vi "RT Accquistion.vi"(7 "Queue ref":T2, 8 "error in":errorcluster, 10 "UI Data":refnum<notifier>, 11 "Task":T3) -> (0 "error out":errorcluster[](array[cluster]))   [LabVIEW 2022 SP3]
uses:
  <vilib>/DAQmx/read.llb/DAQmx Read (Analog 1D Wfm NChan NSamp).vi
  <vilib>/DAQmx/write.llb/DAQmx Write (Analog 1D DBL NChan 1Samp).vi
  <vilib>/DAQmx/write.llb/DAQmx Write (Digital 1D Bool NChan 1Samp 1Line).vi
  <vilib>/DAQmx/read.llb/DAQmx Read (Digital 1D Wfm NChan NSamp).vi
  Source code/Controls/All Loop Status.ctl
  Source code/Controls/All Queue.ctl
  Source code/Controls/UI Data.ctl
panel:
  in  "notification":T1
  out "TC":waveform(dbl)[](array[waveform])
  out "DI":digitalwaveform[](array[waveform])
  out "AI":waveform(dbl)[](array[waveform])
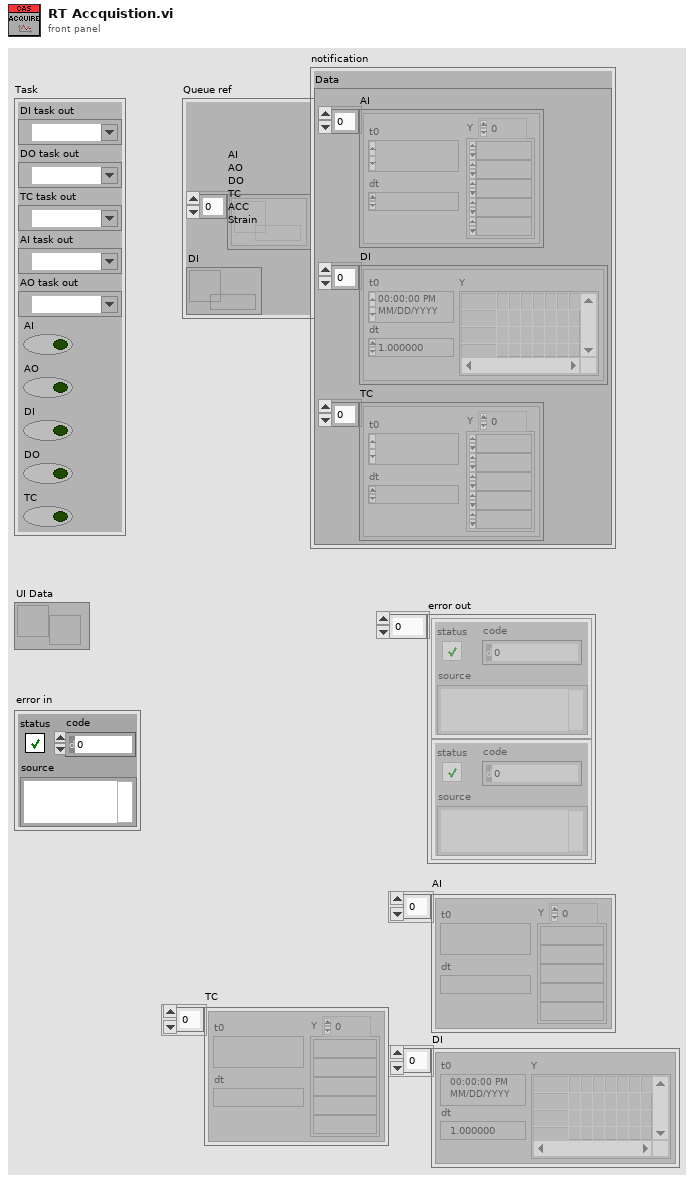
[diagram p1: front panel]
types:
  T1 = typedef "UI Data.ctl" = cluster{"Data":cluster{"AI":waveform(dbl)[], "DI":digitalwaveform[], "TC":waveform(dbl)[]}}
  T2 = typedef "All Queue.ctl" = cluster{"AI\nAO\nDO\nTC\nACC\nStrain":refnum<queue>[], "DI":refnum<queue>}
  T3 = cluster{"DI task out":refnum<k21>, "DO task out":refnum<k21>, "TC task out":refnum<k21>, "AI task out":refnum<k21>, "AO task out":refnum<k21>, "AI":bool, "AO":bool, "DI":bool, "DO":bool, "TC":bool}
  T4 = enum16{"Init", "Read 'All'", "Read 'n'", "Read '1'", "Write '1'", "Write 'n'", "Write 'All'"}
  T5 = typedef "All Loop Status.ctl" = enum16{"AI", "AO", "DI", "DO", "TC", "Strain", "ACC", "RT", "Log"}
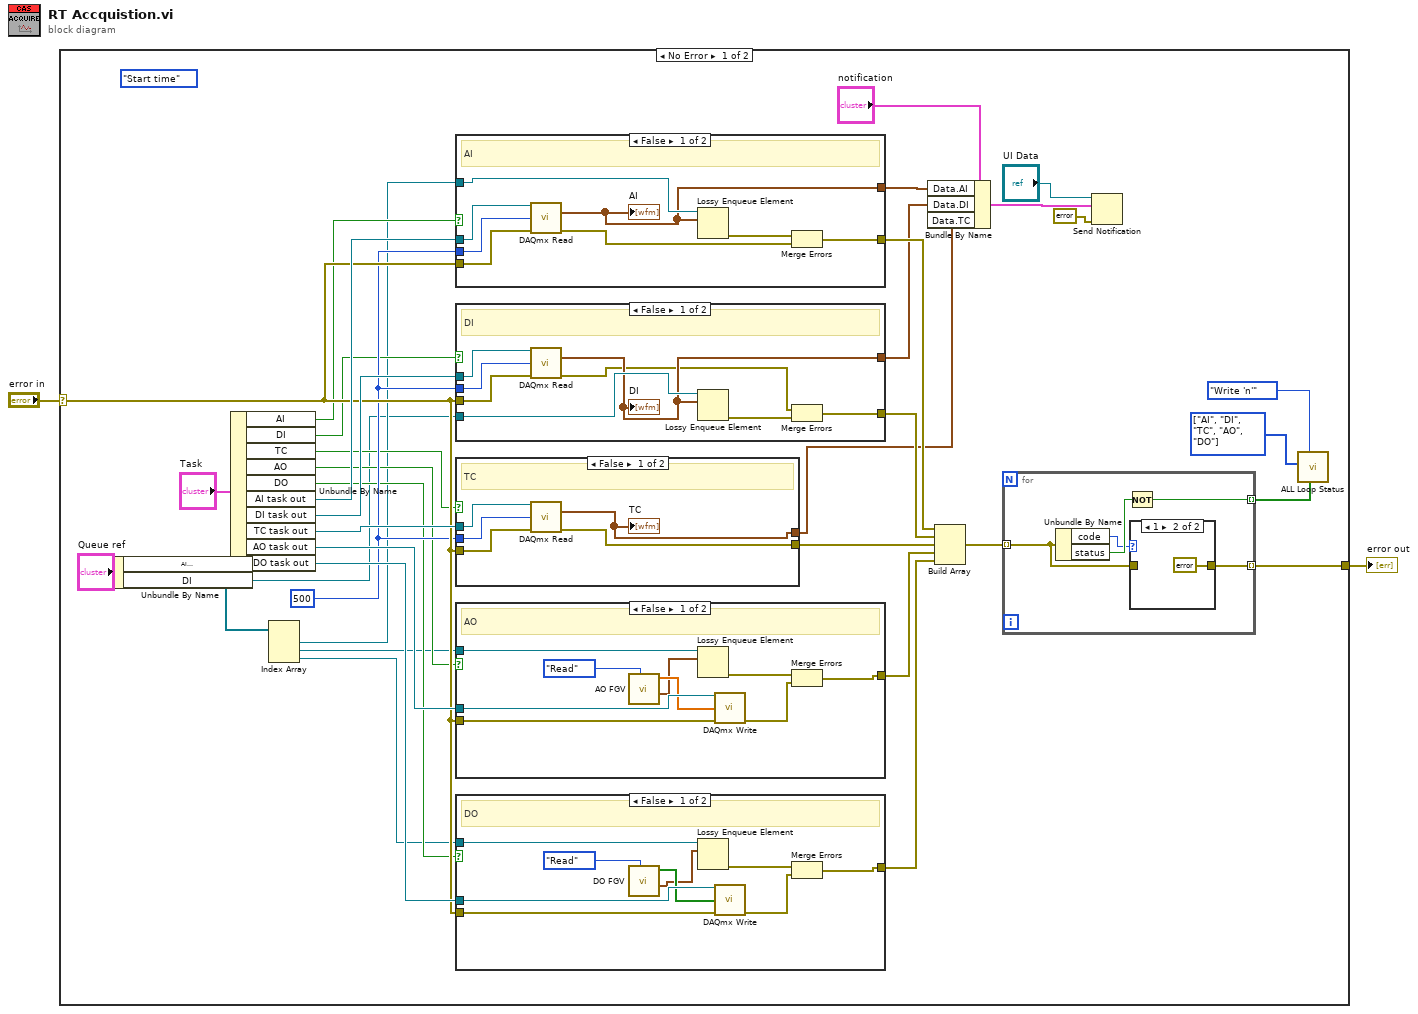
[diagram p0: block diagram]
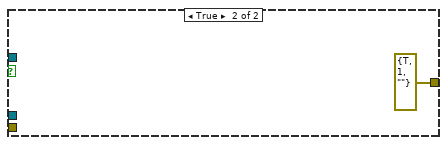
[diagram p3: hidden frame]
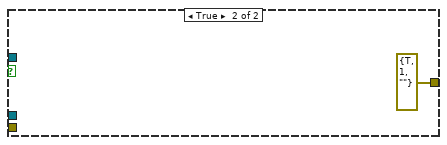
[diagram p4: hidden frame]
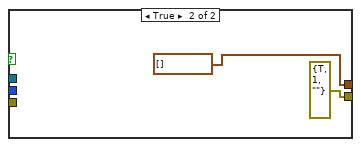
[diagram p5: hidden frame]
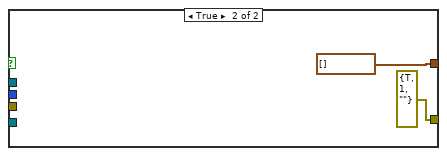
[diagram p6: hidden frame]
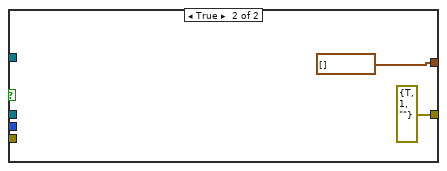
[diagram p7: hidden frame]
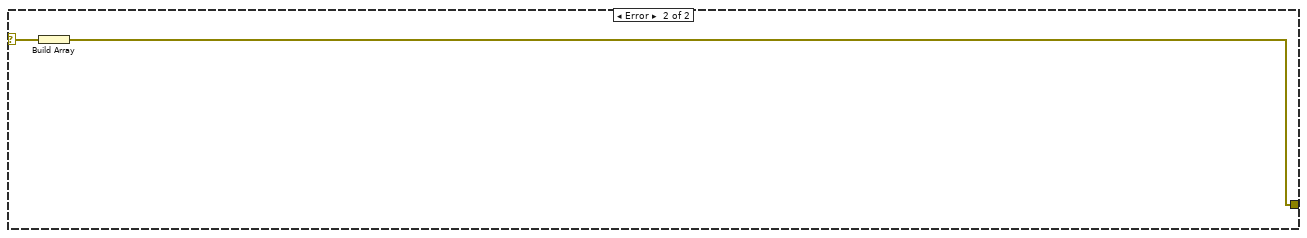
[diagram p8: hidden frame]
diagram:
  n1 = case shown="No Error" "error in" {
    selector: "error in" -> [w28 w94]
    tunnel: [w10 w93] -> w1
    frame No Error {
      (unwired) enum16{"Read", "Write", "Start time", "init"}."Start time" ("Enum")
      w19 = T5[] [enum."AI", enum."DI", enum."TC", enum."AO", enum."DO"] items=["AI", "AO", "DI", "DO", "TC", "Strain", "ACC", "RT", "Log"] ("Loops")
      w27 = 500 ("number of samples per channel")
      n2 = Unbundle By Name("Queue ref") -> ("AI\nAO\nDO\nTC\nACC\nStrain"=w9:refnum<queue>[], "DI"=w6:refnum<queue>)
      n3 = Unbundle By Name("Task") -> ("AI"=w26:bool, "DI"=w25:bool, "TC"=w24:bool, "AO"=w23:bool, "DO"=w22:bool, "AI task out"=w38:refnum<k21>, "DI task out"=w37:refnum<k21>, "TC task out"=w36:refnum<k21>, "AO task out"=w35:refnum<k21>, "DO task out"=w34:refnum<k21>)
      n4 = Index Array(array=w9) -> (element #1=w8:refnum<queue>, element #2=w5:refnum<queue>, element #3=w4:refnum<queue>)  [unwired: 3 in]
      n5 = case shown="False" w26 {
        tunnel: w38 -> [w90 _]
        tunnel: [w85 errorcluster {"status"=TRUE, "code"=1, "source"=""} ("error out")] -> w33
        tunnel: w28 -> [w89 _]
        tunnel: w27 -> [w88 _]
        tunnel: [w83 waveform(dbl)[] [] ("data")] -> w14
        tunnel: w8 -> [w84 _]
        frame False {
          # "AI"
          n6 = call-poly <vilib>:"DAQmx Read.vi"("task/channels in"=w90, "number of samples per channel"=w88, "error in"=w89) -> ("data"=w83:waveform(dbl)[], "error out"=w86:errorcluster)  [unwired: 10 in, 1 out]
          "AI" <- w83
          n7 = Lossy Enqueue Element(queue=w84, element=w83) -> (error out=w87:errorcluster)  [unwired: 1 in, 3 out]
          n8 = Merge Errors(w87, w86) -> (w85:errorcluster)
        }
        frame True {
        }
      }
      n9 = case shown="False" w25 {
        tunnel: w37 -> [w80 _]
        tunnel: [w73 errorcluster {"status"=TRUE, "code"=1, "source"=""} ("error out")] -> w32
        tunnel: w28 -> [w79 _]
        tunnel: w27 -> [w78 _]
        tunnel: [w76 digitalwaveform[] [] ("data")] -> w13
        tunnel: w6 -> [w77 _]
        frame False {
          # "DI"
          n10 = call-poly <vilib>:"DAQmx Read.vi"("task/channels in"=w80, "number of samples per channel"=w78, "error in"=w79) -> ("data"=w76:digitalwaveform[], "error out"=w75:errorcluster)  [unwired: 10 in, 1 out]
          "DI" <- w76
          n11 = Lossy Enqueue Element(queue=w77, element=w76) -> (error out=w74:errorcluster)  [unwired: 1 in, 3 out]
          n12 = Merge Errors(w75, w74) -> (w73:errorcluster)
        }
        frame True {
        }
      }
      n13 = case shown="False" w24 {
        tunnel: w36 -> [w70 _]
        tunnel: [w69 errorcluster {"status"=TRUE, "code"=1, "source"=""} ("error out")] -> w31
        tunnel: w28 -> [w68 _]
        tunnel: w27 -> [w67 _]
        tunnel: [w66 waveform(dbl)[] [] ("data")] -> w12
        frame False {
          # "TC"
          n14 = call-poly <vilib>:"DAQmx Read.vi"("task/channels in"=w70, "number of samples per channel"=w67, "error in"=w68) -> ("data"=w66:waveform(dbl)[], "error out"=w69:errorcluster)  [unwired: 10 in, 1 out]
          "TC" <- w66
        }
        frame True {
        }
      }
      n15 = case shown="False" w23 {
        tunnel: w35 -> [w64 _]
        tunnel: [w61 errorcluster {"status"=TRUE, "code"=1, "source"=""} ("error out")] -> w30
        tunnel: w28 -> [w63 _]
        tunnel: w5 -> [w62 _]
        frame False {
          # "AO"
          n16 = call "AO FGV.vi"("Enum"=enum16{"Read", "Write", "Start time", "init"}."Read") -> ("AO Waveform"=w56:waveform(dbl)[], "AO out"=w58:dbl[])  [unwired: 9 in]
          n17 = Lossy Enqueue Element(queue=w62, element=w56) -> (error out=w60:errorcluster)  [unwired: 1 in, 3 out]
          n18 = call-poly <vilib>:"DAQmx Write.vi"("task/channels in"=w64, "data"=w58, "error in"=w63) -> ("error out"=w59:errorcluster)  [unwired: 10 in, 2 out]
          n19 = Merge Errors(w60, w59) -> (w61:errorcluster)
        }
        frame True {
        }
      }
      n20 = case shown="False" w22 {
        tunnel: w34 -> [w54 _]
        tunnel: [w48 errorcluster {"status"=TRUE, "code"=1, "source"=""} ("error out")] -> w3
        tunnel: w28 -> [w53 _]
        tunnel: w4 -> [w51 _]
        frame False {
          # "DO"
          n21 = call "DO FGV.vi"("Enum"=enum16{"Read", "Write", "Start time", "init"}."Read") -> ("DO Waveform"=w46:waveform(dbl)[], "DO out"=w47:bool[])  [unwired: 9 in]
          n22 = Lossy Enqueue Element(queue=w51, element=w46) -> (error out=w50:errorcluster)  [unwired: 1 in, 3 out]
          n23 = call-poly <vilib>:"DAQmx Write.vi"("task/channels in"=w54, "data"=w47, "error in"=w53) -> ("error out"=w49:errorcluster)  [unwired: 10 in, 2 out]
          n24 = Merge Errors(w50, w49) -> (w48:errorcluster)
        }
        frame True {
        }
      }
      n25 = Bundle By Name(cluster="notification", "Data.AI"=w14, "Data.DI"=w13, "Data.TC"=w12) -> (w16:T1)
      n26 = Build Array(w33, w32, w31, w30, w3) -> (w18:errorcluster[])
      n27 = for {
        tunnel: w18 -> [w39] mode=indexing
        tunnel: [w42] -> w20 mode=indexing
        tunnel: [w40] -> w10 mode=indexing
        n28 = Unbundle By Name(w39) -> ("code"=w41:i32, "status"=w43:bool)
        n29 = Not(x=w43) -> (.not. x?=w42:bool)
        n30 = case shown="1" w41 {
          tunnel: [w44 errorcluster {"status"=FALSE, "code"=0, "source"=""} ("error out")] -> w40
          tunnel: w39 -> [w44 _]
          frame 0, Default {
          }
          frame 1 {
          }
        }
      }
      n31 = Send Notification(notification=w16, notifier="UI Data", error in (no error)=errorcluster {"status"=FALSE, "code"=0, "source"=""}) -> ()  [unwired: 2 out]
      n32 = call "ALL Loop Status.vi"("Status List"=w20, "Option"=T4."Write 'n'", "Loops"=w19) -> ()  [unwired: 6 in, 3 out]
    }
    frame Error {
      n33 = Build Array(w94) -> (w93:errorcluster[])
    }
  }
  "error out" <- w1
